vi "Add Settings.vi"(0 "Configuration Session in":refnum<class "Configuration Session.lvclass">, 1 "id":string, 7 "values":T1, 11 "error in (no error)":errorcluster) -> (4 "Configuration Session out":refnum<class "Configuration Session.lvclass">, 6 "plugin exists?":bool, 15 "error out":errorcluster)   [LabVIEW 2017, in "DSF Core.lvlib" / "Configuration Session.lvclass"]
uses:
  Configuration Session.lvclass
  Typedefs/DSF Settings Info.ctl
  Configuration Session.lvclass/Configuration Session.ctl
  Internal DSF Settings with ID.ctl
  Internal DSF Settings Info.ctl
  DSF Core.lvlib
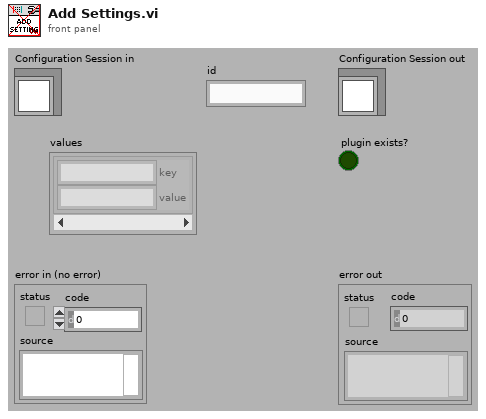
[diagram p1: front panel]
types:
  T1 = typedef "DSF Core.lvlib/DSF Settings Info.ctl" = cluster{"key":string, "value":string}[]
  T2 = typedef "DSF Core.lvlib/Configuration Session.lvclass/Internal DSF Settings with ID.ctl" = cluster{"id":string, "values":T3}
  T3 = typedef "DSF Core.lvlib/Configuration Session.lvclass/Internal DSF Settings Info.ctl" = cluster{"key":string, "value":string}[]
  T4 = typedef "DSF Core.lvlib/Configuration Session.lvclass/DSF Config Data Ref.ctl" = refnum<data-value>
  T5 = typedef "DSF Core.lvlib/Configuration Session.lvclass/DSF Config Data.ctl" = cluster{"dsf configuration":T6, "path":path, "dirty":bool}
  T6 = typedef "DSF Core.lvlib/Configuration Session.lvclass/Internal DSF Configuration.ctl" = cluster{"dsfversion":T7, "version":T7, "plugins":T8[], "groups":T12[], "transfers":T14[], "channels":T16[], "settings":T2[], "framework configuration":T18}
  T7 = typedef "DSF Core.lvlib/DSF Version Info.ctl" = cluster{"major":u32, "minor":u32, "fix":u32, "build":string}
  T8 = typedef "DSF Core.lvlib/Configuration Session.lvclass/Internal DSF Plugin with ID.ctl" = cluster{"id":string, "values":T9}
  T9 = typedef "DSF Core.lvlib/Configuration Session.lvclass/Internal DSF Plugin Info.ctl" = cluster{"components":string[], "timing":T10, "group ids":string[], "settings id":string, "threads":T11[]}
  T10 = typedef "DSF Core.lvlib/DSF Timing Info.ctl" = cluster{"priority":u64, "decimation":u64, "offset":u64}
  T11 = typedef "DSF Core.lvlib/DSF Engine Plugin Thread Configuration.ctl" = cluster{"buffer converter settings":T1, "transceiver settings":T1, "custom settings":T1, "processor":i32, "priority offset":i16}
  T12 = typedef "DSF Core.lvlib/Configuration Session.lvclass/Internal DSF Group with ID.ctl" = cluster{"id":string, "values":T13}
  T13 = typedef "DSF Core.lvlib/Configuration Session.lvclass/Internal DSF Group Info.ctl" = cluster{"direction":i32, "timing":T10, "transfer ids":string[], "settings id":string, "thread":i32, "timeout behavior":u8}
  T14 = typedef "DSF Core.lvlib/Configuration Session.lvclass/Internal DSF Transfer with ID.ctl" = cluster{"id":string, "values":T15}
  T15 = typedef "DSF Core.lvlib/Configuration Session.lvclass/Internal DSF Transfer Info.ctl" = cluster{"byte order":i32, "channel ids":string[], "settings id":string}
  T16 = typedef "DSF Core.lvlib/Configuration Session.lvclass/Internal DSF Channel with ID.ctl" = cluster{"id":string, "values":T17}
  T17 = typedef "DSF Core.lvlib/Configuration Session.lvclass/Internal DSF Channel Info.ctl" = cluster{"string buffer offset":u64, "string data type":i32, "engine data type":i32, "settings id":string, "units":string}
  T18 = typedef "DSF Core.lvlib/DSF Engine Framework Configuration.ctl" = cluster{"Plugins":T19[]}
  T19 = typedef "DSF Core.lvlib/DSF Engine Plugin Configuration.ctl" = cluster{"name":string, "components":string[], "cycle timing":T10, "threads":T11[], "Transfer Groups":T20[], "settings":T1}
  T20 = typedef "DSF Core.lvlib/DSF Engine Transfer Group Configuration.ctl" = cluster{"name":string, "direction":T21, "cycle timing":T10, "thread index":i32, "settings":T1, "Transfers":T22[], "timeout behavior":T26}
  T21 = typedef "DSF Core.lvlib/DSF Direction.ctl" = enum8{"Tx", "Rx"}
  T22 = typedef "DSF Core.lvlib/DSF Engine Transfer Configuration.ctl" = cluster{"name":string, "byte order":T23, "settings":T1, "channels":T24[]}
  T23 = typedef "DSF Core.lvlib/DSF Byte Order.ctl" = enum8{"big-endian", "little-endian"}
  T24 = typedef "DSF Core.lvlib/DSF Engine Channel Configuration.ctl" = cluster{"string offset":u64, "string data type":T25, "engine data type":T25, "name":string, "settings":T1, "units":string}
  T25 = typedef "DSF Core.lvlib/DSF Data Type.ctl" = enum8{"Bool", "SGL", "DBL", "I8", "I16", "I32", "I64", "U8", "U16", "U32", "U64"}
  T26 = typedef "DSF Core.lvlib/DSF Timeout Behavior.ctl" = enum8{"Increment Late Count", "Throw Error"}
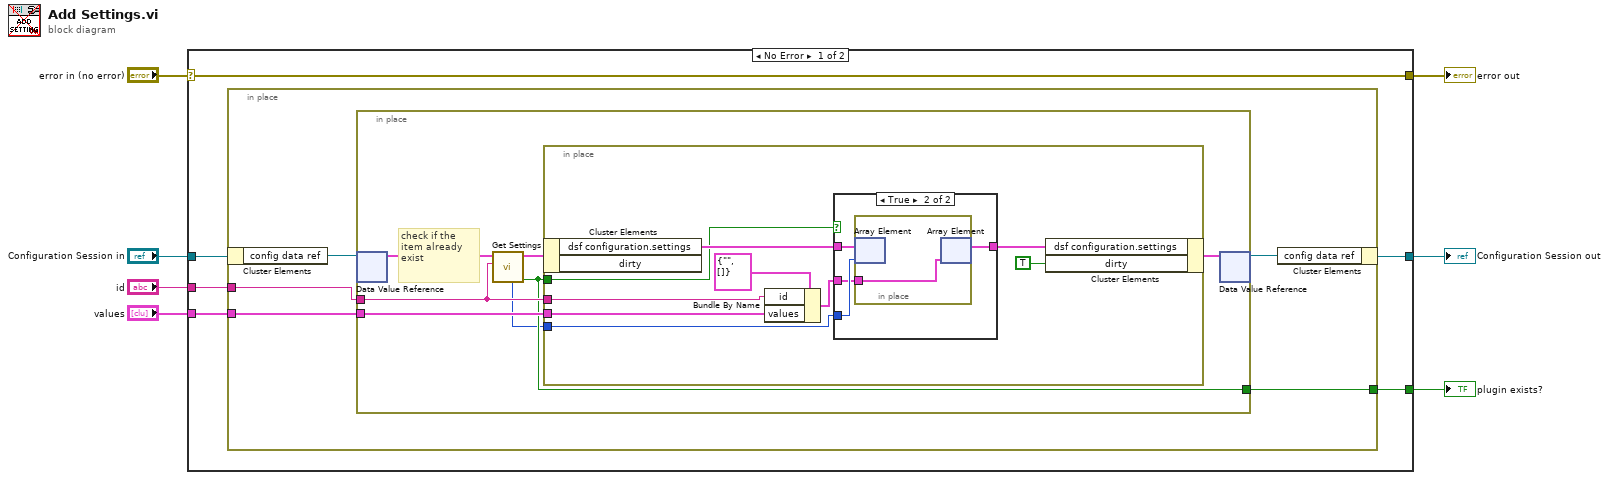
[diagram p0: block diagram]
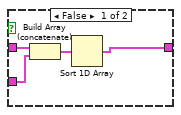
[diagram p2: hidden frame]
diagram:
  n1 = case shown="No Error" "error in (no error)" {
    selector: "error in (no error)" -> [w13 w45]
    tunnel: [w13 w45] -> w6
    tunnel: [w8 w44] -> w1
    tunnel: "Configuration Session in" -> [w9 w44]
    tunnel: "id" -> [w12 _]
    tunnel: "values" -> [w11 _]
    tunnel: [w10 _] -> w3
    frame No Error {
      n2 = in-place {
        in-place-border: w12 -> [w18]
        in-place-border: w11 -> [w17]
        in-place-border: [w16] -> w10
        n3 = in-place-cluster #1(w9) -> ("config data ref"=w15:T4)
        n4 = in-place {
          in-place-border: w18 -> [w25]
          in-place-border: w17 -> [w23]
          in-place-border: [w22] -> w16
          # "check if the item already exist"
          n5 = in-place-dvr #2(w15) -> (w19:T5)  [unwired: 1 out]
          n6 = call "Get Settings.vi"("id"=w25, "DSF Configuration in"=w19) -> ("exists?"=w22:bool, "DSF Configuration out"=w24:T5, "index"=w21:i32)  [unwired: 6 in, 1 out]
          n7 = in-place {
            in-place-border: w25 -> [w33]
            in-place-border: w23 -> [w31]
            in-place-border: w22 -> [w30]
            in-place-border: w21 -> [w29]
            n8 = in-place-cluster #3(w24) -> ("dsf configuration.settings"=w34:T2[])  [unwired: 1 out]
            n9 = Bundle By Name(cluster=T2 {"id"="", "values"=[]} ("settings"), "id"=w33, "values"=w31) -> (w27:T2)
            n10 = case shown="True" w30 {
              tunnel: w34 -> [w38 w42]
              tunnel: [w37 w39] -> w32
              tunnel: w29 -> [_ w41]
              tunnel: w27 -> [w35 w40]
              frame False {
                n11 = Build Array (concatenate)(w38, w35) -> (w36:T2[])
                n12 = Sort 1D Array(array=w36) -> (sorted array=w37:T2[])
              }
              frame True {
                n13 = in-place {
                  in-place-border: w40 -> [w43]
                  n14 = in-place-array #4(w42, w41) -> ()  [unwired: 1 out]
                  n15 = in-place-array #4(w43) -> (w39:T2[])  [unwired: 1 out]
                }
              }
            }
            n16 = in-place-cluster #3("dsf configuration.settings"=w32, "dirty"=TRUE) -> (w20:T5)
          }
          n17 = in-place-dvr #2(w20) -> (w14:T4)  [unwired: 1 out]
        }
        n18 = in-place-cluster #1("config data ref"=w14) -> (w8:refnum<class "Configuration Session.lvclass">)
      }
    }
    frame Error {
    }
  }
  "error out" <- w6
  "plugin exists?" <- w3
  "Configuration Session out" <- w1
